vi "initImages.vi"() -> (3 "output cluster":T1)   [LabVIEW 2013]
uses:
  analysis_data_typdef.ctl
  IMAQ Image.ctl
  MagAnalysis_Online.lvclass
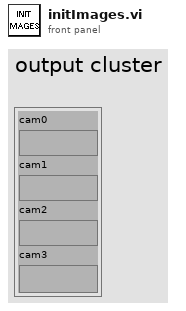
[diagram p1: front panel]
types:
  T1 = typedef "MagAnalysis_Online.lvclass/analysis_data_typdef.ctl" = cluster{"cam0":T2, "cam1":T2, "cam2":T2, "cam3":T2}
  T2 = typedef "IMAQ Image.ctl" = refnum<image>
  T3 = typedef "Image Type" = u32
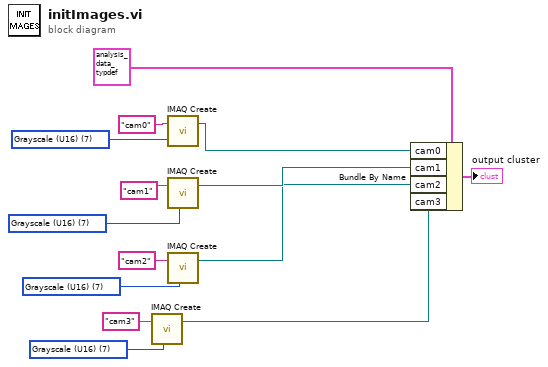
[diagram p0: block diagram]
diagram:
  w8 = T3 7 items=["Grayscale (U8)", "Grayscale (I16)", "Grayscale (SGL)", "Complex (CSG)", "RGB (U32)", "HSL (U32)", "RGB (U64)", "Grayscale (U16)"] ("Image Type")
  w9 = T3 7 items=["Grayscale (U8)", "Grayscale (I16)", "Grayscale (SGL)", "Complex (CSG)", "RGB (U32)", "HSL (U32)", "RGB (U64)", "Grayscale (U16)"] ("Image Type")
  w12 = T3 7 items=["Grayscale (U8)", "Grayscale (I16)", "Grayscale (SGL)", "Complex (CSG)", "RGB (U32)", "HSL (U32)", "RGB (U64)", "Grayscale (U16)"] ("Image Type")
  w13 = T3 7 items=["Grayscale (U8)", "Grayscale (I16)", "Grayscale (SGL)", "Complex (CSG)", "RGB (U32)", "HSL (U32)", "RGB (U64)", "Grayscale (U16)"] ("Image Type")
  n1 = call "IMAQ Create"("Image Name"="cam3", "Image Type"=w8) -> ("New Image"=w2:T2)  [unwired: 3 in, 1 out]
  n2 = call "IMAQ Create"("Image Name"="cam0", "Image Type"=w13) -> ("New Image"=w5:T2)  [unwired: 3 in, 1 out]
  n3 = call "IMAQ Create"("Image Name"="cam1", "Image Type"=w12) -> ("New Image"=w4:T2)  [unwired: 3 in, 1 out]
  n4 = call "IMAQ Create"("Image Name"="cam2", "Image Type"=w9) -> ("New Image"=w3:T2)  [unwired: 3 in, 1 out]
  n5 = Bundle By Name(cluster=T1 {"cam0"=refnum, "cam1"=refnum, "cam2"=refnum, "cam3"=refnum} ("data 2"), "cam0"=w5, "cam1"=w4, "cam2"=w3, "cam3"=w2) -> (→"output cluster":T1)
